vi "Remove illegal file characters.vi"(11 "Filename In":string) -> (3 "Filename Out":string)   [LabVIEW 2013]
uses:
  <vilib>/regexp/Match Regular Expression.xnode
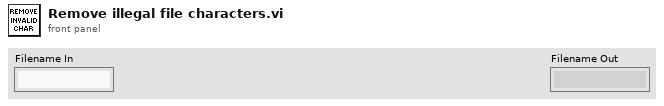
[diagram p1: front panel]
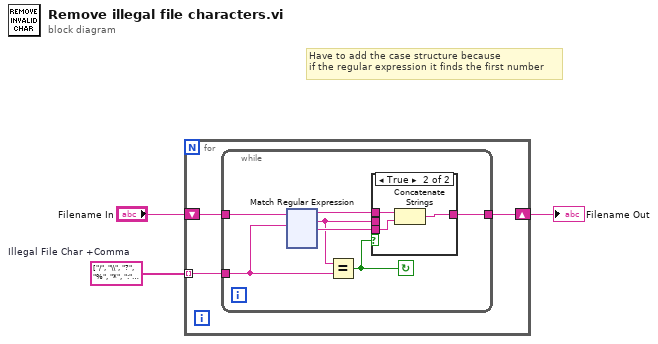
[diagram p0: block diagram]
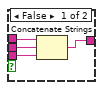
[diagram p2: hidden frame]
diagram:
  w1 = string[] ["/", "\\", "?", "%", "*", ":", "|", "\"", "<", ">", ".", ","]  # Illegal File Char +Comma
  # "Have to add the case structure because\nif the regular expression it finds the first number"
  n1 = for {
    shift-right: [w4] -> w3
    shift-left: "Filename In" -> [w5]
    tunnel: w1 -> [w6] mode=indexing
    n2 = while {
      tunnel: w6 -> [w9]
      tunnel: w5 -> [w13]
      tunnel: [w10] -> w4
      stop <- w8 continue-if-true
      n3 = xnode "Match Regular Expression"("input string"=w13, "regular expression"=w9) -> ("before match"=w12:string, "whole match"=w7:string, "after match"=w11:string)  [unwired: 4 in, 2 out]
      n4 = Equal?(x=w7, y=w9) -> (x = y?=w8:bool)
      n5 = case shown="True" w8 {
        tunnel: w12 -> [w16 w20]
        tunnel: w11 -> [w17 w19]
        tunnel: [w15 w18] -> w10
        tunnel: w7 -> [w14 _]
        frame False {
          n6 = Concatenate Strings(w16, w14, w17) -> (w15:string)
        }
        frame True {
          n7 = Concatenate Strings(w20, w19) -> (w18:string)
        }
      }
    }
  }
  "Filename Out" <- w3
